vi "add_CMDMPC.vi"(6 "MPC Info":T1 {"c"."3" format="%#_12g"; "c"."2" format="%#_12g"; "c"."1" format="%#_12g"}, 7 "msg in":string) -> (3 "msg out":string)   [LabVIEW 2018]
doc: "Flattens a pose 2D into a message"
uses:
  <userlib>/ROS for LabVIEW Software/ROS/MessageBuilding/std_msgs/subs/float64Scalar.vi
  <userlib>/ROS for LabVIEW Software/ROS/MessageBuilding/std_msgs/subs/i32Scalar.vi
  <userlib>/ROS for LabVIEW Software/ROS/MessageBuilding/std_msgs/subs/float64Array.vi
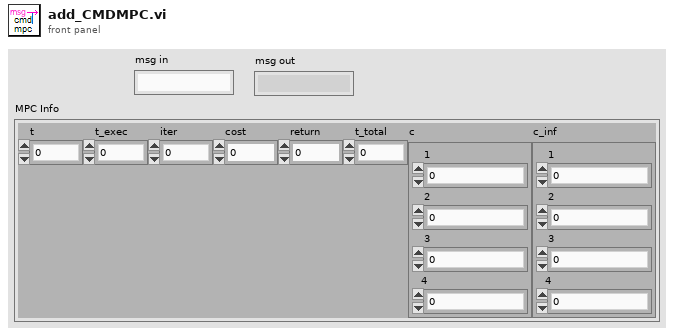
[diagram p1: front panel]
types:
  T1 = cluster{"t":dbl, "t_exec":dbl, "iter":i32, "cost":dbl, "return":i32, "t_total":dbl, "c":cluster{"1":dbl, "2":dbl, "3":dbl, "4":dbl}, "c_inf":cluster{"1":dbl, "2":dbl, "3":dbl, "4":dbl}}
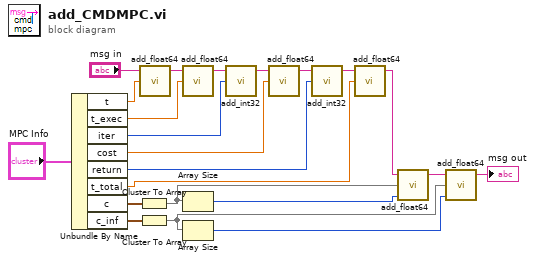
[diagram p0: block diagram]
diagram:
  n1 = Unbundle By Name("MPC Info") -> ("t"=w14:dbl, "t_exec"=w15:dbl, "iter"=w16:i32, "cost"=w17:dbl, "return"=w18:i32, "t_total"=w19:dbl, "c"=w21:cluster{"1":dbl, "2":dbl, "3":dbl, "4":dbl}, "c_inf"=w20:cluster{"1":dbl, "2":dbl, "3":dbl, "4":dbl})
  n2 = Cluster To Array(cluster=w21) -> (array=w2:dbl[])
  n3 = Cluster To Array(cluster=w20) -> (array=w4:dbl[])
  n4 = call-poly <userlib>:"add_float64.vi"("Numeric"=w14, "msg in"="msg in") -> ("msg out"=w12:string)  [unwired: 3 in]
  n5 = call-poly <userlib>:"add_float64.vi"("Numeric"=w15, "msg in"=w12) -> ("msg out"=w11:string)  [unwired: 3 in]
  n6 = Array Size(array=w2) -> (size(s)=w1:i32)
  n7 = Array Size(array=w4) -> (size(s)=w3:i32)
  n8 = call-poly "add_int32.vi"("Numeric"=w16, "msg in"=w11) -> ("msg out"=w10:string)  [unwired: 3 in]
  n9 = call-poly <userlib>:"add_float64.vi"("Numeric"=w17, "msg in"=w10) -> ("msg out"=w9:string)  [unwired: 3 in]
  n10 = call-poly "add_int32.vi"("Numeric"=w18, "msg in"=w9) -> ("msg out"=w8:string)  [unwired: 3 in]
  n11 = call-poly <userlib>:"add_float64.vi"("Numeric"=w19, "msg in"=w8) -> ("msg out"=w7:string)  [unwired: 3 in]
  n12 = call-poly <userlib>:"add_float64.vi"("Array Length"=w1, "Array"=w2, "msg in"=w7) -> ("msg out"=w6:string)  [unwired: 2 in]
  n13 = call-poly <userlib>:"add_float64.vi"("Array Length"=w3, "Array"=w4, "msg in"=w6) -> ("msg out"=→"msg out":string)  [unwired: 2 in]
